vi "Enable or Disable Modem Status Controls.vi"(11 "error in (no error)":errorcluster) -> (15 "error out":errorcluster)   [LabVIEW 2011]
doc: "This VI enables or disables the PCP controls based on the digital values that are read. The disable property nodes will not be written unless the condition for disabling/enabling has been changed."
uses:
  Measurments Handling/Status Digitalish.ctl
  Controll refrence groups.ctl
  Modem Status/Variable List Modem Status Digital.ctl
  emi Lib/Basic/1 - GUI/Control tools/Private/emi_Control enable and visibility array.vi
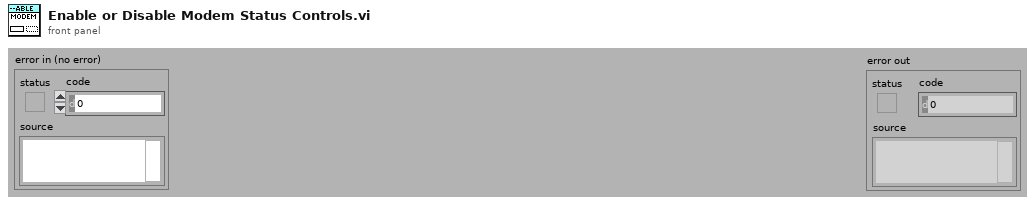
[diagram p1: front panel]
types:
  T1 = typedef "Variable List Modem Status Digital.ctl" = enum16{"TMU_LINK_STATUS"}
  T2 = typedef "Controll refrence groups.ctl" = enum16{"Controller. gen", "Controller . High G", "Stroker", "PCP Online", "PCP Local", "PCP HV On", "Driller", "Stroker Cmd Buttons", "Stroker Anchor Cmd Buttons", "Controller Relay Buttons", "PCP Start Telemetry", "PCP Start Motor", "Tractor", "Modem Status"}
  T3 = typedef "Status Digitalish.ctl" = enum16{"NA", "False", "True"}
  T4 = cluster{"Controll collection":T2, bool, "State(Normal)":enum16{"Normal", "Disabled", "Grayed", "Hidden"}}
  T5 = cluster{"Controll collection":T2, bool, "State(Normal)":enum16{"Normal", "Disabled", "Grayed", "Hidden"}}[]
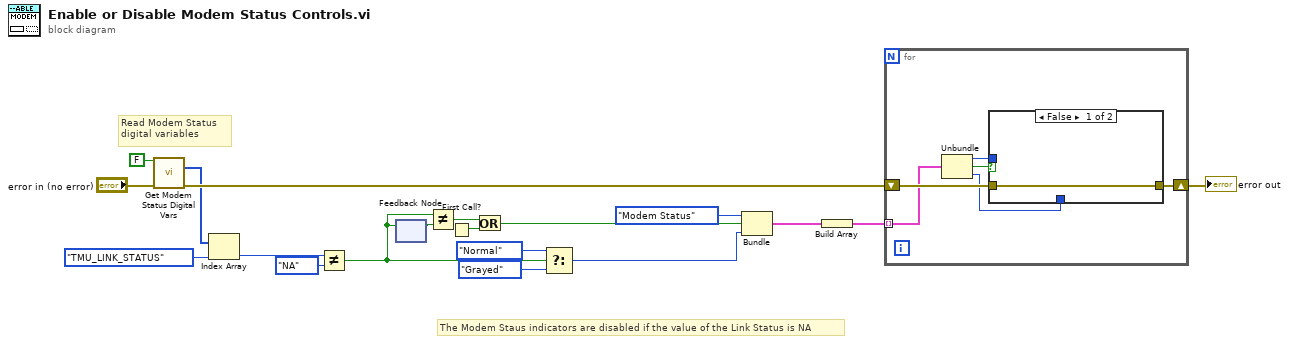
[diagram p0: block diagram]
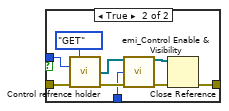
[diagram p2: hidden frame]
diagram:
  # "Read Modem Status \ndigital variables"
  # "The Modem Staus indicators are disabled if the value of the Link Status is NA"
  n1 = call "Get Modem Status Digital Vars.vi"("Common alarm handling(F)"=FALSE, "error in (no error)"="error in (no error)") -> ("Values"=w2:T3[], "error out"=w3:errorcluster)  [unwired: 7 in, 5 out]
  n2 = Index Array(array=w2, index=Variable_List_Modem_Status_Digital."TMU_LINK_STATUS" ("Enum")) -> (element=w17:T3)
  n3 = Not Equal?(x=w17, y=Status_Digitalish."NA") -> (x != y?=w6:bool)
  n4 = feedback #1() -> (w15:bool)  [unwired: 1 in]
  n5 = feedback-in #1(w6) -> ()
  n6 = Not Equal?(x=w6, y=w15) -> (x != y?=w13:bool)
  n7 = First Call?() -> (First Call?: T/F=w14:bool)
  n8 = Or(x=w13, y=w14) -> (x .or. y?=w12:bool)
  n9 = Select(t=enum16{"Normal", "Disabled", "Grayed", "Hidden"}."Normal" ("State(Normal)"), s=w6, f=enum16{"Normal", "Disabled", "Grayed", "Hidden"}."Grayed" ("State(Normal)")) -> (s? t:f=w10:enum16{"Normal", "Disabled", "Grayed", "Hidden"})
  n10 = Bundle("Controll collection"=Controll_refrence_groups."Modem Status", w12, "State(Normal)"=w10) -> (w9:T4)  [unwired: 1 in]
  n11 = Build Array(w9) -> (w8:T5)
  n12 = for {
    tunnel: w8 -> [w24] mode=indexing
    shift-right: [w20] -> w7
    shift-left: w3 -> [w25]
    n13 = Unbundle(w24) -> ("Controll collection"=w23:T2, w22:bool, "State(Normal)"=w21:enum16{"Normal", "Disabled", "Grayed", "Hidden"})
    n14 = case shown="False" w22 {
      tunnel: w25 -> [w26 w31]
      tunnel: [w26 w30] -> w20
      tunnel: w23 -> [_ w29]
      tunnel: w21 -> [_ w28]
      frame False {
      }
      frame True {
        n15 = call "Control refrence holder.vi"("Action(GET)"=enum16{"GET", "SET"}."GET", "Controll collection"=w29, "error in (no error)"=w31) -> ("Controlls out"=w35:refnum<vi>[], "error out"=w34:errorcluster)  [unwired: 11 in]
        n16 = call-poly "emi_Control Enable & Visibility.vi"("Controls"=w35, "State(Normal)"=w28, "error in"=w34) -> ("Constrols out"=w32:refnum<vi>[], "error out"=w33:errorcluster)  [unwired: 11 in]
        n17 = Close Reference(reference=w32, error in (no error)=w33) -> (error out=w30:errorcluster)
      }
    }
  }
  "error out" <- w7
